vi "DFIR End Run.vi"(0 "Numeric":dbl) -> ()   [LabVIEW 2011]
panel:
  out "Waveform Chart":dbl(graph)
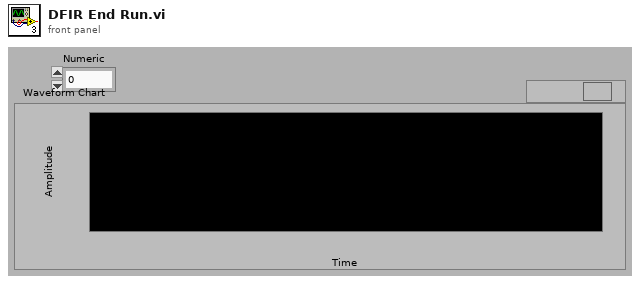
[diagram p1: front panel]
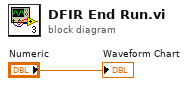
[diagram p0: block diagram]
diagram:
  "Waveform Chart" <- "Numeric"
